vi "emi_Error Finder.vi"   [LabVIEW 2010]
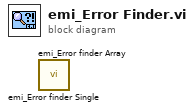
[diagram p0: block diagram]
diagram:
  n1 = call "emi_Error finder Single.vi"() -> ()  [unwired: 12 in, 4 out]
  n2 = call "emi_Error finder Array.vi"() -> ()  [unwired: 12 in, 4 out]
